vi "Get Meta File Name.vi"(0 "Base Path":path, 5 "Bridge":string="a", 7 "cRIO":string="a", 9 "Impact Location":i32, 11 "Average Number":i32) -> (4 "Full Path":path)   [LabVIEW 2012]
panel:
  out "Result Filename":string
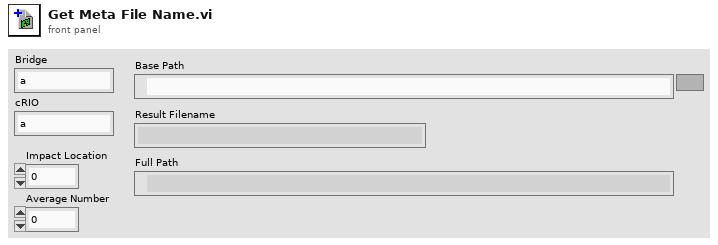
[diagram p1: front panel]
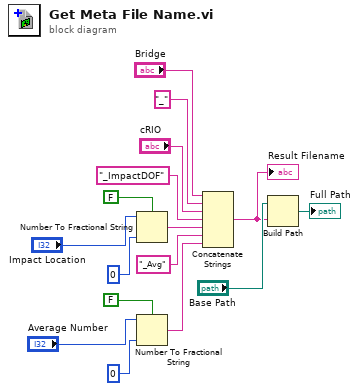
[diagram p0: block diagram]
diagram:
  n1 = Number To Fractional String(use system decimal point (T)=FALSE, number="Impact Location", precision (6)=i16 0) -> (F-format string=w6:string)  [unwired: 1 in]
  n2 = Number To Fractional String(use system decimal point (T)=FALSE, number="Average Number", precision (6)=i16 0) -> (F-format string=w4:string)  [unwired: 1 in]
  n3 = Concatenate Strings("Bridge", "_", "cRIO", "_ImpactDOF", w6, "_Avg", w4) -> (w9:string)
  "Result Filename" <- w9
  n4 = Build Path(base path="Base Path", name or relative path=w9) -> (appended path=→"Full Path":path)
